vi "RadarPlot.vi"() -> ()   [LabVIEW 2009]
panel:
  out "Radar Plot":picture
  in  "Column Header":string
  in  "Row Header":string
  in  "Columns":i32
  in  "Rows":i32
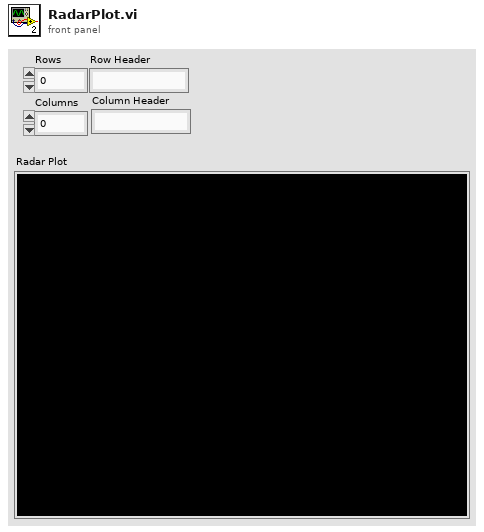
[diagram p1: front panel]
types:
  T1 = cluster{"color (white)":u32, "format and precision":cluster{"format":enum8{"Decimal", "Scientific", "Engineering", "Binary", "Octal", "Hex"}, "precision":u8}, "autoscale? (false)":bool}
  T2 = cluster{"position (none)":enum16{"none", "top", "right", "bottom", "left"}, "text color(white)":u32}
  T3 = typedef "LVBoundsTypeDef.ctl" = cluster{"Width":u32, "Height":u32}
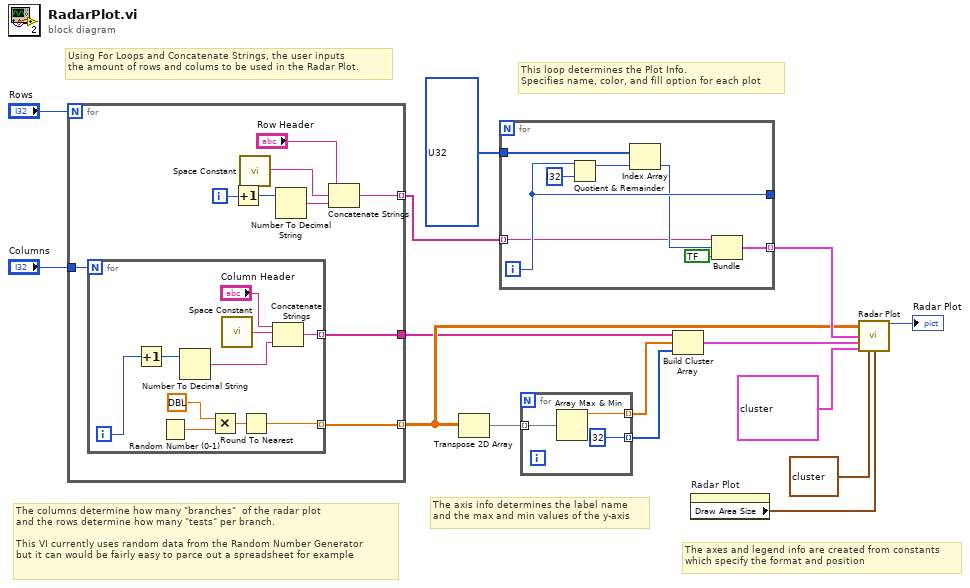
[diagram p0: block diagram]
diagram:
  # "The axis info determines the label name \nand the max and min values of the y-axis"
  # "The axes and legend info are created from constants\nwhich specify the format and position"
  # "This loop determines the Plot Info. \nSpecifies name, color, and fill option for each plot"
  # "The columns determine how many \"branches\"  of the radar plot\nand the rows determine how many \"tests\" per branch. \n\nThis VI currently uses random data from the Random Number Generator\nbut it can would be fairly easy to parce out a spreadsheet for example"
  # "Using For Loops and Concatenate Strings, the user inputs\nthe amount of rows and colums to be used in the Radar Plot."
  n1 = for {
    N: "Rows" -> [_]
    tunnel: "Columns" -> [w24]
    tunnel: [w18] -> w9 mode=indexing
    tunnel: [w17] -> w8
    tunnel: [w16] -> w11 mode=indexing
    i -> [w19]
    n2 = for {
      N: w24 -> [_]
      tunnel: [w27] -> w18 mode=indexing
      tunnel: [w26] -> w17 mode=indexing
      i -> [w25]
      n3 = Increment(x=w25) -> (x+1=w34:i32)
      n4 = Random Number (0-1)() -> (number: 0 to 1=w29:dbl)
      n5 = Number To Decimal String(number=w34) -> (decimal integer string=w33:string)  [unwired: 1 in]
      n6 = Multiply(x=dbl ?, y=w29) -> (x*y=w30:dbl)
      n7 = call <vilib>:"Space Constant.vi"() -> ("String"=w32:string)
      n8 = Round To Nearest(number=w30) -> (nearest integer value=w27:dbl)
      n9 = Concatenate Strings("Column Header", w32, w33) -> (w26:string)
    }
    n10 = Increment(x=w19) -> (x+1=w20:i32)
    n11 = call <vilib>:"Space Constant.vi"() -> ("String"=w21:string)
    n12 = Number To Decimal String(number=w20) -> (decimal integer string=w23:string)  [unwired: 1 in]
    n13 = Concatenate Strings("Row Header", w21, w23) -> (w16:string)
  }
  n14 = Transpose 2D Array(2D array=w9) -> (transposed array=w13:dbl[][])
  n15 = for {
    tunnel: [w42] -> _
    tunnel: u32[] ? -> [w41]
    tunnel: w11 -> [w37] mode=indexing
    tunnel: [w35] -> w10 mode=indexing
    i -> [w42]
    n16 = Quotient & Remainder(x=w42, y=i32 ?) -> (x-y*floor(x/y)=w39:i32)  [unwired: 1 out]
    n17 = Index Array(array=w41, index=w39) -> (element=w38:u32)
    n18 = Bundle(w37, w38, bool ?) -> (w35:cluster{string, u32, bool})  [unwired: 1 in]
  }
  n19 = for {
    tunnel: w13 -> [w45] mode=indexing
    tunnel: [w44] -> w7 mode=indexing
    tunnel: [i32 ?] -> w6 mode=indexing
    n20 = Array Max & Min(array=w45) -> (max value=w44:dbl)  [unwired: 3 out]
  }
  n21 = Build Cluster Array(w8, w7, w6) -> (w5:cluster{string, dbl, i32}[])
  n22 = property on="Radar Plot" class="Pict"() -> ("Draw Area Size"=w3:T3)  [unwired: 2 in, 2 out]
  n23 = call <vilib>:"Radar Plot.vi"("data"=w9, "plot info"=w10, "axis info"=w5, "axes info"=T1 ?, "legend info"=T2 ?, "dimension (w,h)"=w3) -> ("new picture"=→"Radar Plot":picture)  [unwired: 9 in]
